vi "Teleop.vi"(10 "Match Info":T1={"Autonomous Elapsed Seconds"=0.0, "TeleOp Elapsed Seconds"=0.0, "Disabled Elapsed Seconds"=0.0, "Visited Autonomous"=FALSE, "Visited TeleOp"=FALSE, "Visited Disabled"=FALSE, "Autonomous Settings"={"Autonomous Style"=enum."Independent", "VI Refnum"=refnum}}, 11 "Call Context":T2) -> ()   [LabVIEW 2015]
doc: "This VI is called for each TeleOp packet received from the DS where the robot is not disabled. It is often used to read from the joysticks and update I/O or to update setpoints for timed control loops. It should complete and return within 20 milliseconds or it may miss DS packets."
uses:
  <vilib>/Rock Robotics/WPI/DriverStation/WPI_DriverStationDerivedRobotMode.ctl
  <vilib>/Rock Robotics/WPI/DriverStation/WPI_DriverStationMatch Info.ctl
  <vilib>/Rock Robotics/WPI/Utilities/WPI_GetSetVariantRefNum.vi
  <vilib>/Rock Robotics/Network Tables/NT Read Number.vi
  <vilib>/Rock Robotics/Network Tables/NT Write Boolean Array.vi
  <vilib>/Rock Robotics/Network Tables/NT Write Numeric Array.vi
  <vilib>/Rock Robotics/Network Tables/NT Read Boolean.vi
  <vilib>/Rock Robotics/Network Tables/NT Write Number.vi
panel:
  in  "Feeder Speed":dbl=-100.0
  out "Position Control":dbl
  in  "Intake Speed":dbl=-30.0 format="%#_13g"
  out "Sample Slider 0":dbl(slide) scale=0.0..5.0
  out "Sample Boolean 1":bool
  out "Sample Boolean 0":bool
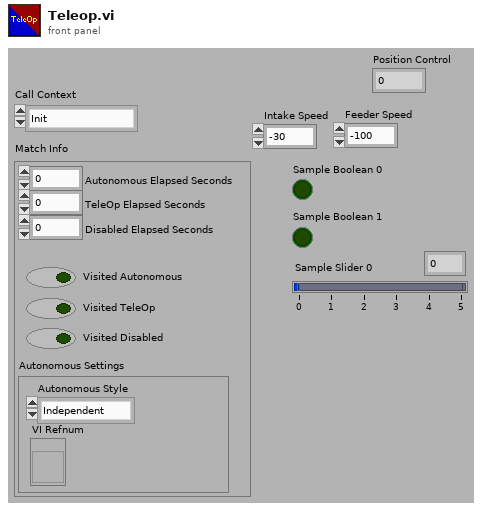
[diagram p1: front panel]
types:
  T1 = typedef "WPI_DriverStationMatch Info.ctl" = cluster{"Autonomous Elapsed Seconds":dbl, "TeleOp Elapsed Seconds":dbl, "Disabled Elapsed Seconds":dbl, "Visited Autonomous":bool, "Visited TeleOp":bool, "Visited Disabled":bool, "Autonomous Settings":cluster{"Autonomous Style":enum16{"Iterative", "Independent"}, "VI Refnum":refnum<vi>}}
  T2 = typedef "WPI_DriverStationDerivedRobotMode.ctl" = enum16{"Init", "Execute", "Stop"}
  T3 = typedef "WPI_JoystickDevRef.ctl" = cluster{"Device":T4}
  T4 = typedef "WPI_JoystickDeviceEnum.ctl" = enum16{"USB 0", "USB 1", "USB 2", "USB 3", "USB 4", "USB 5"}
  T5 = typedef "WPI_MotorControlDeviceRef.ctl" = cluster{"DeviceStatus":errorcluster, "Type":T6, "PWM":cluster{"PWM Channel":T7, "DeadBand":T8}, "CAN":cluster{"Device Number":u8, "Control Mode":T9, "Semaphore":T10, "Max Vout":dbl, "TalonSRX Control Mode":T11}, "Invert":bool}
  T6 = typedef "WPI_MotorControlType.ctl" = enum16{"PWM", "CAN", "CANTalonSRX"}
  T7 = typedef "FPGA_DIOPWMChannel.ctl" = enum8{"PWM 0", "PWM 1", "PWM 2", "PWM 3", "PWM 4", "PWM 5", "PWM 6", "PWM 7", "PWM 8", "PWM 9", "PWM MXP 0", "PWM MXP 1", "PWM MXP 2", "PWM MXP 3", "PWM MXP 4", "PWM MXP 5", "PWM MXP 6", "PWM MXP 7", "PWM MXP 8", "PWM MXP 9", "Invalid"}
  T8 = typedef "WPI_PWMDeadband.ctl" = cluster{"Name":string, "maxPositivePwm":i32, "minPositivePwm":i32, "centerPwm":i32, "maxNegativePwm":i32, "minNegativePwm":i32, "angularRange":u16}
  T9 = typedef "WPI_CANJaguar_ControlMode.ctl" = enum8{"Percent VBus", "Current", "Speed", "Position", "Voltage"}
  T10 = typedef "Semaphore RefNum" = refnum<k1>
  T11 = typedef "WPI_CANTalonSRX_APIControlMode.ctl" = enum8{"Percent VBus", "Speed", "Position", "Slave", "Unchanged / Invalid", "Voltage Compensation", "Current", "Motion Profile"}
  T12 = cluster{"LeftX":dbl, "LeftY":dbl, "LTrigger":dbl, "RTrigger":dbl, "RightX":dbl, "RightY":dbl, "RightY 2":dbl, "RightX 2":dbl}
  T13 = cluster{"ButtonA":bool, "ButtonB":bool, "ButtonX":bool, "ButtonY":bool, "ButtonLB":bool, "ButtonRB":bool, "ButtonBack":bool, "ButtonStart":bool, "Button1":bool, "Button2":bool}
  T14 = typedef "WPI_RobotDriveDevRef.ctl" = cluster{"DevStatus":errorcluster, "Motors[]":T5[], "Square Inputs":bool, "Max Output":dbl}
  T15 = typedef "WPI_DigitalInputDevRef.ctl" = cluster{"DevStatus":errorcluster, "DIO Channel":T16}
  T16 = typedef "FPGA_DIOChannel.ctl" = enum8{"DIO 0", "DIO 1", "DIO 2", "DIO 3", "DIO 4", "DIO 5", "DIO 6", "DIO 7", "DIO 8", "DIO 9", "DIO MXP 0", "DIO MXP 1", "DIO MXP 2", "DIO MXP 3", "DIO MXP 4", "DIO MXP 5", "DIO MXP 6", "DIO MXP 7", "DIO MXP 8", "DIO MXP 9", "DIO MXP 10", "DIO MXP 11", "DIO MXP 12", "DIO MXP 13", "DIO MXP 14", "DIO MXP 15", "Invalid"}
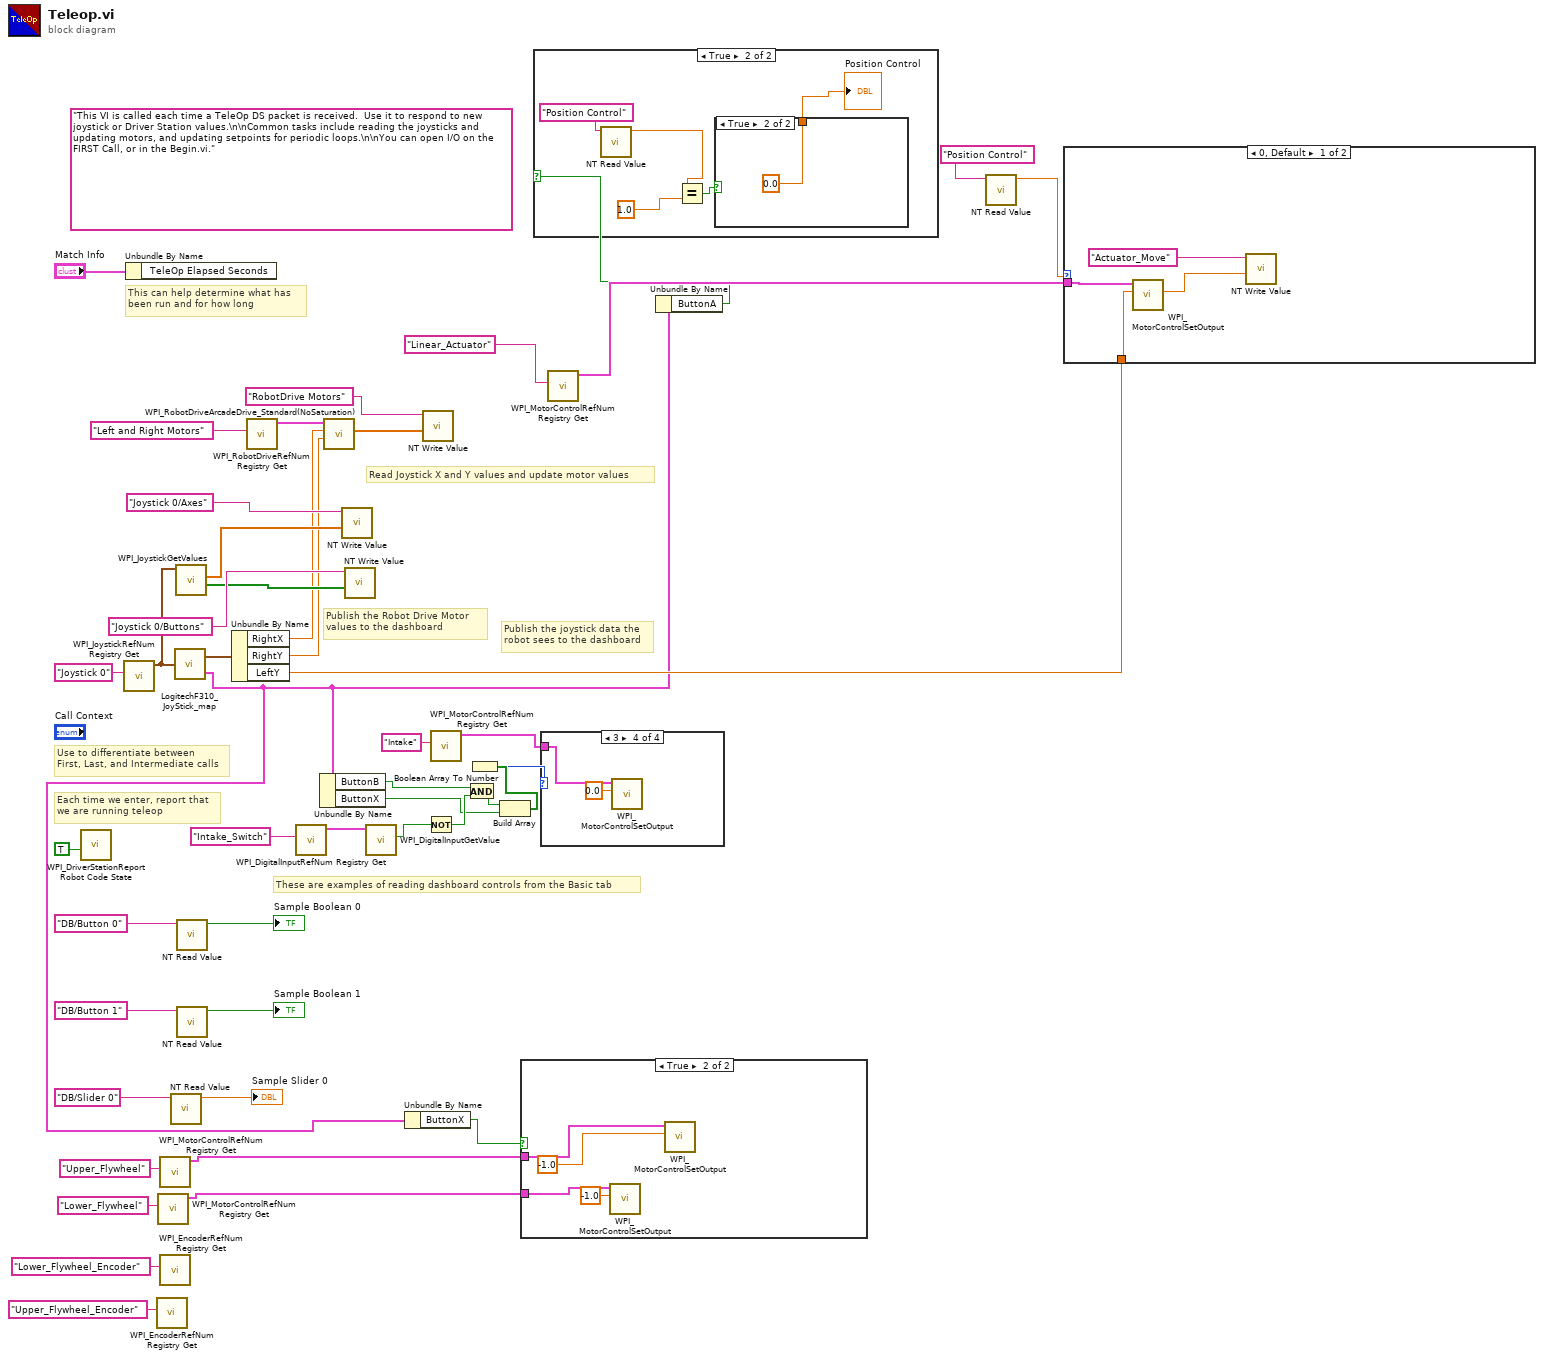
[diagram p0: block diagram]
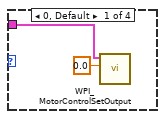
[diagram p2: hidden frame]
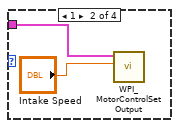
[diagram p3: hidden frame]
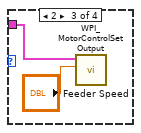
[diagram p4: hidden frame]
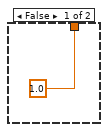
[diagram p6: hidden frame]
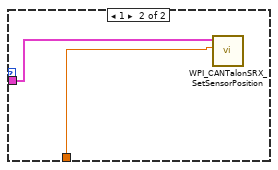
[diagram p7: hidden frame]
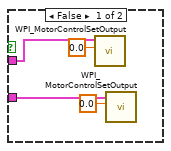
[diagram p8: hidden frame]
diagram:
  (unwired) "This VI is called each time a TeleOp DS packet is received.  Use it to respond to new joystick or Driver Station values.\n\nCommon tasks include reading the joysticks and updating motors, and updating setpoints for periodic loops.\n\nYou can open I/O on the FIRST Call, or in the Begin.vi."
  # "These are examples of reading dashboard controls from the Basic tab"
  # "Publish the Robot Drive Motor\nvalues to the dashboard"
  # "Publish the joystick data the\nrobot sees to the dashboard"
  # "Each time we enter, report that\nwe are running teleop"
  # "Use to differentiate between\nFirst, Last, and Intermediate calls"
  # "This can help determine what has\nbeen run and for how long"
  # "Read Joystick X and Y values and update motor values"
  n1 = call <vilib>:"WPI_DriverStationReport Robot Code State.vi"("TeleOp"=TRUE ("Autonomous")) -> ()  [unwired: 10 in, 1 out]
  n2 = call <vilib>:"WPI_JoystickRefNum Registry Get.vi"("refnum name"="Joystick 0") -> ("JoystickDevRef"=w25:T3)  [unwired: 1 in, 9 out]
  n3 = Unbundle By Name("Match Info") -> ()  [unwired: 1 out]
  n4 = call <vilib>:"WPI_EncoderRefNum Registry Get.vi"("refnum name"="Upper_Flywheel_Encoder") -> ()  [unwired: 9 in, 2 out]
  n5 = call <vilib>:"WPI_MotorControlRefNum Registry Get.vi"("refnum name"="Lower_Flywheel") -> ("MotorControlDevRef"=w17:T5)  [unwired: 9 in, 1 out]
  n6 = call <vilib>:"WPI_MotorControlRefNum Registry Get.vi"("refnum name"="Upper_Flywheel") -> ("MotorControlDevRef"=w18:T5)  [unwired: 9 in, 1 out]
  n7 = call <vilib>:"WPI_EncoderRefNum Registry Get.vi"("refnum name"="Lower_Flywheel_Encoder") -> ()  [unwired: 9 in, 2 out]
  n8 = call-poly <vilib>:"NT Read Value.vi"("Name"="DB/Slider 0" ("refnum name")) -> ("Numeric"=→"Sample Slider 0":dbl)  [unwired: 9 in, 1 out]
  n9 = call "LogitechF310_JoyStick_map.vi"("JoystickDevRef"=w25) -> ("AxesCluster"=w29:T12, "ButtonsCluster"=w16:T13)
  n10 = call <vilib>:"WPI_JoystickGetValues.vi"("JoystickDevRef"=w25) -> ("Buttons"=w38:bool[], "Axes"=w39:dbl[])  [unwired: 6 in, 3 out]
  n11 = call-poly <vilib>:"NT Read Value.vi"("Name"="DB/Button 0" ("refnum name")) -> ("Boolean"=→"Sample Boolean 0":bool)  [unwired: 9 in, 1 out]
  n12 = call-poly <vilib>:"NT Read Value.vi"("Name"="DB/Button 1" ("refnum name")) -> ("Boolean"=→"Sample Boolean 1":bool)  [unwired: 9 in, 1 out]
  n13 = Unbundle By Name(w29) -> ("RightX"=w28:dbl, "RightY"=w27:dbl, "LeftY"=w23:dbl)
  n14 = call <vilib>:"WPI_RobotDriveRefNum Registry Get.vi"("refnum name"="Left and Right Motors") -> ("RobotDriveDevRef"=w44:T14)  [unwired: 1 in, 9 out]
  n15 = call <vilib>:"WPI_DigitalInputRefNum Registry Get.vi"("refnum name"="Intake_Switch") -> ("DigitalInputDevRef"=w12:T15)  [unwired: 9 in, 1 out]
  n16 = Unbundle By Name(w16) -> ("ButtonB"=w10:bool, "ButtonX"=w5:bool)
  n17 = call <vilib>:"WPI_RobotDriveArcadeDrive_Standard(NoSaturation).vi"("Y axis value"=w27, "X axis value"=w28, "RobotDriveDevRef"=w44) -> ("Motor Values"=w31:dbl[])  [unwired: 1 in, 7 out]
  n18 = call-poly <vilib>:"NT Write Value.vi"("Numeric Array"=w39, "Name"="Joystick 0/Axes") -> ()  [unwired: 9 in, 1 out]
  n19 = call-poly <vilib>:"NT Write Value.vi"("Boolean Array"=w38, "Name"="Joystick 0/Buttons") -> ()  [unwired: 9 in, 1 out]
  n20 = call <vilib>:"WPI_DigitalInputGetValue.vi"("DigitalInputDevRef"=w12) -> ("Value"=w8:bool)  [unwired: 8 in, 2 out]
  n21 = Unbundle By Name(w16) -> ("ButtonX"=w21:bool)
  n22 = call-poly <vilib>:"NT Write Value.vi"("Numeric Array"=w31, "Name"="RobotDrive Motors") -> ()  [unwired: 9 in, 1 out]
  n23 = Not(x=w8) -> (.not. x?=w11:bool)
  n24 = call <vilib>:"WPI_MotorControlRefNum Registry Get.vi"("refnum name"="Intake") -> ("MotorControlDevRef"=w7:T5)  [unwired: 9 in, 1 out]
  n25 = And(x=w10, y=w11) -> (x .and. y?=w6:bool)
  n26 = Build Array(w6, w5) -> (w4:bool[])
  n27 = Boolean Array To Number(Boolean array=w4) -> (number=w3:u32)
  n28 = case shown="True" w21 {
    tunnel: w18 -> [w49 w54]
    tunnel: w17 -> [w50 w53]
    frame False {
      n29 = call <vilib>:"WPI_MotorControlSetOutput.vi"("Output"=0.0, "MotorControlDevRef"=w49) -> ()  [unwired: 7 in, 3 out]
      n30 = call <vilib>:"WPI_MotorControlSetOutput.vi"("Output"=0.0, "MotorControlDevRef"=w50) -> ()  [unwired: 7 in, 3 out]
    }
    frame True {
      n31 = call <vilib>:"WPI_MotorControlSetOutput.vi"("Output"=-1.0, "MotorControlDevRef"=w53) -> ()  [unwired: 7 in, 3 out]
      n32 = call <vilib>:"WPI_MotorControlSetOutput.vi"("Output"=-1.0, "MotorControlDevRef"=w54) -> ()  [unwired: 7 in, 3 out]
    }
  }
  n33 = case shown="3" w3 {
    tunnel: w7 -> [w55 w57 w60 w62]
    frame 0, Default {
      n34 = call <vilib>:"WPI_MotorControlSetOutput.vi"("Output"=0.0, "MotorControlDevRef"=w55) -> ()  [unwired: 7 in, 3 out]
    }
    frame 1 {
      n35 = call <vilib>:"WPI_MotorControlSetOutput.vi"("Output"="Intake Speed", "MotorControlDevRef"=w57) -> ()  [unwired: 7 in, 3 out]
    }
    frame 2 {
      n36 = call <vilib>:"WPI_MotorControlSetOutput.vi"("Output"="Feeder Speed", "MotorControlDevRef"=w60) -> ()  [unwired: 7 in, 3 out]
    }
    frame 3 {
      n37 = call <vilib>:"WPI_MotorControlSetOutput.vi"("Output"=0.0, "MotorControlDevRef"=w62) -> ()  [unwired: 7 in, 3 out]
    }
  }
  n38 = call <vilib>:"WPI_MotorControlRefNum Registry Get.vi"("refnum name"="Linear_Actuator") -> ("MotorControlDevRef"=w24:T5)  [unwired: 9 in, 1 out]
  n39 = Unbundle By Name(w16) -> ("ButtonA"=w15:bool)
  n40 = case shown="True" w15 {
    frame False {
    }
    frame True {
      n41 = call-poly <vilib>:"NT Read Value.vi"("Name"="Position Control") -> ("Numeric"=w64:dbl)  [unwired: 9 in, 1 out]
      n42 = Equal?(x=w64, y=1.0) -> (x = y?=w66:bool)
      n43 = case shown="True" w66 {
        tunnel: [1.0 ("Position Control") 0.0 ("Position Control")] -> w63
        frame False {
        }
        frame True {
        }
      }
      "Position Control" <- w63
    }
  }
  n44 = call-poly <vilib>:"NT Read Value.vi"("Name"="Position Control") -> ("Numeric"=w13:dbl)  [unwired: 9 in, 1 out]
  n45 = case shown="0, Default" w13 {
    tunnel: w24 -> [w70 w75]
    tunnel: w23 -> [w71 w74]
    frame 0, Default {
      n46 = call <vilib>:"WPI_MotorControlSetOutput.vi"("Output"=w71, "MotorControlDevRef"=w70) -> ("Motor Output"=w73:dbl)  [unwired: 7 in, 2 out]
      n47 = call-poly <vilib>:"NT Write Value.vi"("Numeric"=w73, "Name"="Actuator_Move") -> ()  [unwired: 9 in, 1 out]
    }
    frame 1 {
      n48 = call <vilib>:"WPI_CANTalonSRX_SetSensorPosition.vi"("New Sensor Position"=w74, "CAN Talon SRX Ref"=w75) -> ()  [unwired: 8 in, 2 out]
    }
  }
